vi "Pre Launch Init.vi"(11 "Mag Lab Measure Base in":refnum<class "Mag Lab Measure Base.lvclass">) -> (0 "error out":errorcluster, 3 "Mag Lab Measure Base out":refnum<class "Mag Lab Measure Base.lvclass">)   [LabVIEW 2015, in "Mag Lab Measure Base.lvclass"]
doc: "(<B>Filename</B>: Actor Framework.lvlib:Actor.lvclass:Pre Launch Init.vi)\n\nDefines behavior that occurs after the Launch Actor method is invoked but before the actor's Actor Core method begins running.\n\nThe Pre Launch Init method is guaranteed to finish before the Launch Actor method returns to its caller and before the actor itself receives any messages. Any references that the Pre Launch Init method obtains are guaranteed to have the same lifetime as the actor itself. Any errors that the Pre Launch Init method returns will abort the launch.\n\nBy default, this method does nothing. A descendant class may override it to define behavior."
uses:
  Mag Lab Measure Base.lvclass
  Mag Lab Measure Base.lvclass/Mag Lab Measure Base.ctl
  Mag Lab Root/Mag Lab Root.lvclass
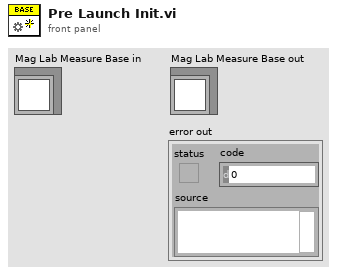
[diagram p1: front panel]
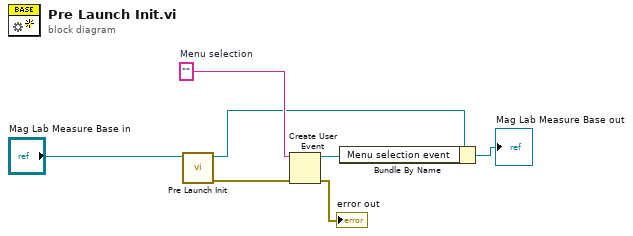
[diagram p0: block diagram]
diagram:
  w6 = ""  # Menu selection
  n1 = call-parent "Pre Launch Init.vi"("Mag Lab Root in"="Mag Lab Measure Base in") -> ("error out"=w1:errorcluster, "Mag Lab Root out"=w4:refnum<class "Mag Lab Measure Base.lvclass">)  [unwired: 9 in]
  n2 = Create User Event(user event datatype=w6, error in=w1) -> (user event=w5:refnum<user-event>, error out=→"error out":errorcluster)
  n3 = Bundle By Name(cluster=w4, "Menu selection event"=w5) -> (→"Mag Lab Measure Base out":refnum<class "Mag Lab Measure Base.lvclass">)
